vi "List Mode - Set Configurations for Program Setup.vi"   [LabVIEW 2014, in "Associated Power Technologies 8500 Series.lvlib"]
uses:
  <instrlib>/Associated Power Technologies 8500 Series/Associated Power Technologies 8500 Series.lvlib
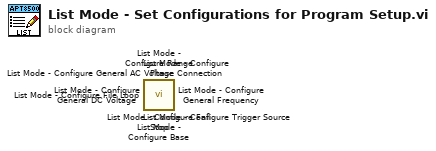
[diagram p0: block diagram]
diagram:
  n1 = call <instrlib>:"List Mode - Configure Fail Stop.vi"() -> ()  [unwired: 10 in, 2 out]
  n2 = call <instrlib>:"List Mode - Configure Phase Connection.vi"() -> ()  [unwired: 10 in, 2 out]
  n3 = call <instrlib>:"List Mode - Configure General DC Voltage.vi"() -> ()  [unwired: 10 in, 2 out]
  n4 = call <instrlib>:"List Mode - Configure General Frequency.vi"() -> ()  [unwired: 10 in, 2 out]
  n5 = call <instrlib>:"List Mode - Configure General AC Voltage.vi"() -> ()  [unwired: 10 in, 2 out]
  n6 = call <instrlib>:"List Mode - Configure Range.vi"() -> ()  [unwired: 10 in, 2 out]
  n7 = call <instrlib>:"List Mode - Configure Base.vi"() -> ()  [unwired: 10 in, 2 out]
  n8 = call <instrlib>:"List Mode - Configure Trigger Source.vi"() -> ()  [unwired: 10 in, 2 out]
  n9 = call <instrlib>:"List Mode - Configure File Loop.vi"() -> ()  [unwired: 10 in, 2 out]
